vi "Quadratic Function.vi"(1 "x":refnum<class "Dual.lvclass">) -> (0 "f(x)":refnum<class "Dual.lvclass">)   [LabVIEW 2020, in "Examples.lvlib"]
doc: "f(x) = (x-3)^2"
uses:
  classes/Dual/Dual.lvclass
  classes/Dual/Dual.lvclass/Dual.ctl
  01818c0d-791c-47f2-b729-6465b175f802.vi
  c3e93b09-8303-4840-bc75-75d53694f5a4.vi
  066be19f-15d0-4b13-ac21-78bd1faad0bc.vi
  01818c0d-791c-47f2-b729-6465b175f802.vi/5957e011-cf56-4527-b6ed-13c3a4ca997b.vi
  classes/Dual/Write a.vi
  c3e93b09-8303-4840-bc75-75d53694f5a4.vi/968883c3-f1f3-473a-bfc5-8cde3e5b01f7.vi
  c3e93b09-8303-4840-bc75-75d53694f5a4.vi/bec82738-76c0-439a-a1c7-54fdd631a6e8.vi
  classes/Dual/Read a and b.vi
  classes/Dual/Write a and b.vi
  066be19f-15d0-4b13-ac21-78bd1faad0bc.vi/957074e8-cc3b-4647-8ff1-d975a744cd4e.vi
  Examples.lvlib
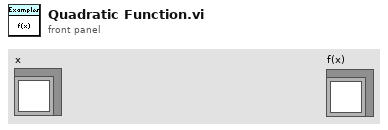
[diagram p1: front panel]
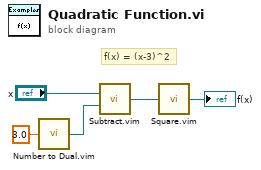
[diagram p0: block diagram]
diagram:
  # "f(x) = (x-3)^2"
  n1 = call "Number to Dual.vim"("Number"=3.0 ("Double")) -> ("Dual"=w2:refnum<class "Dual.lvclass">)
  n2 = call "Subtract.vim"("x"="x", "y"=w2) -> ("x - y"=w3:refnum<class "Dual.lvclass">)  [unwired: 13 in]
  n3 = call "Square.vim"("x"=w3) -> ("x^2"=→"f(x)":refnum<class "Dual.lvclass">)
